vi "Activate Masters.vi"(8 "error in (no error)":errorcluster, 11 "BME_DG_System in":refnum<class "BME_DG_System.lvclass">) -> (0 "error out":errorcluster, 3 "BME_DG_System out":refnum<class "BME_DG_System.lvclass">)   [LabVIEW 2009, in "POLARIS BME DG.lvlib" / "BME_DG_System.lvclass"]
uses:
  BME_DG_System.lvclass
  BME_DG_System.lvclass/BME_DG_System.ctl
  BME_DG_Base/BME_DG_Base.lvclass
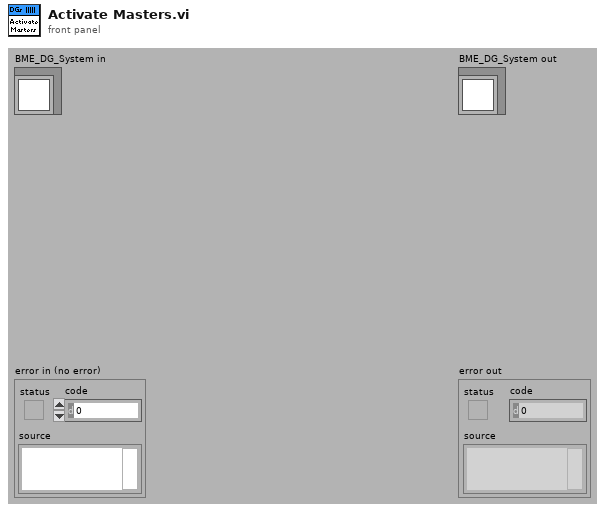
[diagram p1: front panel]
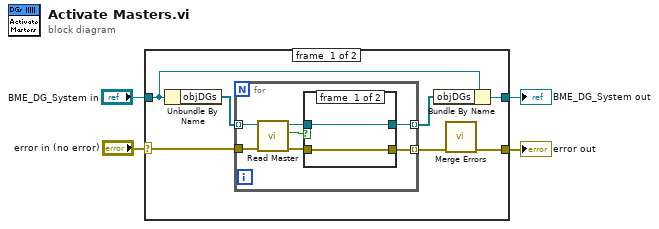
[diagram p0: block diagram]
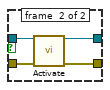
[diagram p2: hidden frame]
diagram:
  n1 = case shown="No Error" "error in (no error)" {
    selector: "error in (no error)" -> [w9 w26]
    tunnel: [w5 w26] -> w3
    tunnel: [w8 w25] -> w1
    tunnel: "BME_DG_System in" -> [w11 w25]
    frame #0 {
      n2 = Unbundle By Name(w11) -> ("objDGs"=w10:refnum<class "BME_DG_Base.lvclass">[])
      n3 = for {
        tunnel: w10 -> [w16] mode=indexing
        tunnel: w9 -> [w14]
        tunnel: [w18] -> w6 mode=indexing
        tunnel: [w17] -> w7 mode=indexing
        n4 = call-dynamic "Read Master.vi"("error in (no error)"=w14, "BME_DG_Base in"=w16) -> ("error out"=w13:errorcluster, "Master?"=w12:bool, "BME_DG_Base out"=w15:refnum<class "BME_DG_Base.lvclass">)  [unwired: 6 in, 1 out]
        n5 = case shown="True" w12 {
          tunnel: w15 -> [w20 w24]
          tunnel: w13 -> [w19 w23]
          tunnel: [w19 w22] -> w18
          tunnel: [w20 w21] -> w17
          frame #0 {
          }
          frame #1 {
            n6 = call-dynamic "Activate.vi"("error in (no error)"=w23, "BME_DG_Base in"=w24) -> ("error out"=w22:errorcluster, "BME_DG_Base out"=w21:refnum<class "BME_DG_Base.lvclass">)  [unwired: 8 in]
          }
        }
      }
      n7 = Bundle By Name(cluster=w11, "objDGs"=w7) -> (w8:refnum<class "BME_DG_System.lvclass">)
      n8 = call <vilib>:"Merge Errors.vi"("error array in"=w6) -> ("error out"=w5:errorcluster)  [unwired: 6 in]
    }
    frame #1 {
    }
  }
  "error out" <- w3
  "BME_DG_System out" <- w1
